vi "Set Temperature.vi"(8 "error in (no error)":errorcluster, 11 "CCDCamera in":refnum<class "Real Camera.lvclass">) -> (0 "error out":errorcluster, 3 "CCDCamera out":refnum<class "Real Camera.lvclass">)   [LabVIEW 2018, in "Real Camera.lvclass"]
doc: "Set the CCD temperature"
uses:
  Real Camera.lvclass
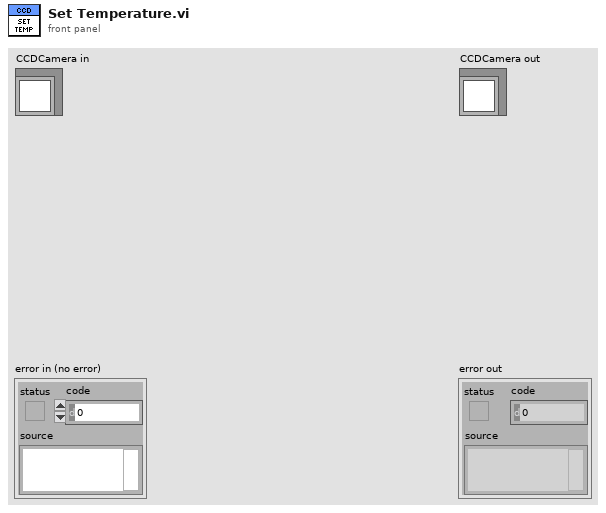
[diagram p1: front panel]
types:
  T1 = cluster{"COOLER_POWER_STATUS":u16, "TEMP":i32, "EXPTIME":dbl, "#FRAMES":u32}
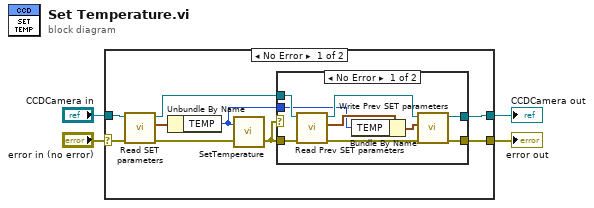
[diagram p0: block diagram]
diagram:
  n1 = case shown="No Error" "error in (no error)" {
    selector: "error in (no error)" -> [w13 w25]
    tunnel: "CCDCamera in" -> [w11 w26]
    tunnel: [w10 w26] -> w1
    tunnel: [w9 w25] -> w4
    frame No Error {
      n2 = call-dynamic "Read SET parameters.vi"("error in (no error)"=w13, "Simulated_CCD_Camera in"=w11) -> ("error out"=w5:errorcluster, "New SET parameters"=w12:T1, "Simulated_CCD_Camera out"=w7:refnum<class "Real Camera.lvclass">)  [unwired: 7 in]
      n3 = Unbundle By Name(w12) -> ("TEMP"=w8:i32)
      n4 = call <userlib>:"SetTemperature.vi"("error in (no error)"=w5, "temperature"=w8) -> ("error out"=w6:errorcluster)  [unwired: 1 out]
      n5 = case shown="No Error" w6 {
        tunnel: [w22 w24] -> w10
        tunnel: [w21 w23] -> w9
        tunnel: w7 -> [w17 w24]
        tunnel: w6 -> [w18 w23]
        tunnel: w8 -> [w14 _]
        frame No Error {
          n6 = call-dynamic "Read Prev SET parameters.vi"("error in (no error)"=w18, "Simulated_CCD_Camera in"=w17) -> ("error out"=w19:errorcluster, "Prev SET parameters"=w16:T1, "Simulated_CCD_Camera out"=w20:refnum<class "Real Camera.lvclass">)  [unwired: 7 in]
          n7 = Bundle By Name(cluster=w16, "TEMP"=w14) -> (w15:T1)
          n8 = call-dynamic "Write Prev SET parameters.vi"("error in (no error)"=w19, "Prev SET parameters"=w15, "Simulated_CCD_Camera in"=w20) -> ("error out"=w21:errorcluster, "Simulated_CCD_Camera out"=w22:refnum<class "Real Camera.lvclass">)  [unwired: 7 in]
        }
        frame Error {
        }
      }
    }
    frame Error {
    }
  }
  "error out" <- w4
  "CCDCamera out" <- w1
